vi "Set Control Appearance.vi"(4 "DigNum Refnum 2":refnum<vi>, 5 "DigNum Refnum":refnum<vi>, 6 "Bool Refnum":refnum<vi>, 7 "Arr Refnum":refnum<vi>, 8 "error in (no error)":errorcluster, 9 "Slide Refnum":refnum<vi>, 10 "Data In":T3, 11 "Display State In":T2 caption="State" {"# of Loops" min=1 step=1; "Index" min=0 step=1; "Program"."Step" min=0.001 max=80.0 step=0.001 format="%.2f"; "Program"."Target" format="%.2f"}) -> (0 "error out":errorcluster, 2 "Data Out":T3 caption="Data In", 3 "Display State Out":T2 caption="State" {"# of Loops" min=1 step=1; "Index" min=0 step=1; "Program"."Step" min=0.001 max=80.0 step=0.001 format="%.2f"; "Program"."Target" format="%.2f"})   [LabVIEW 2012, in "Multi Segment Waveform.xctl"]
doc: "Based on the current XControl state, set the appearance of the facade controls"
uses:
  Multi Segment Waveform.xctl
  State.ctl
  Data.ctl
  <vilib>/_xctls/Container State.ctl
  <vilib>/_xctls/XControlSupport.lvlib
panel:
  in  "Container State":T1
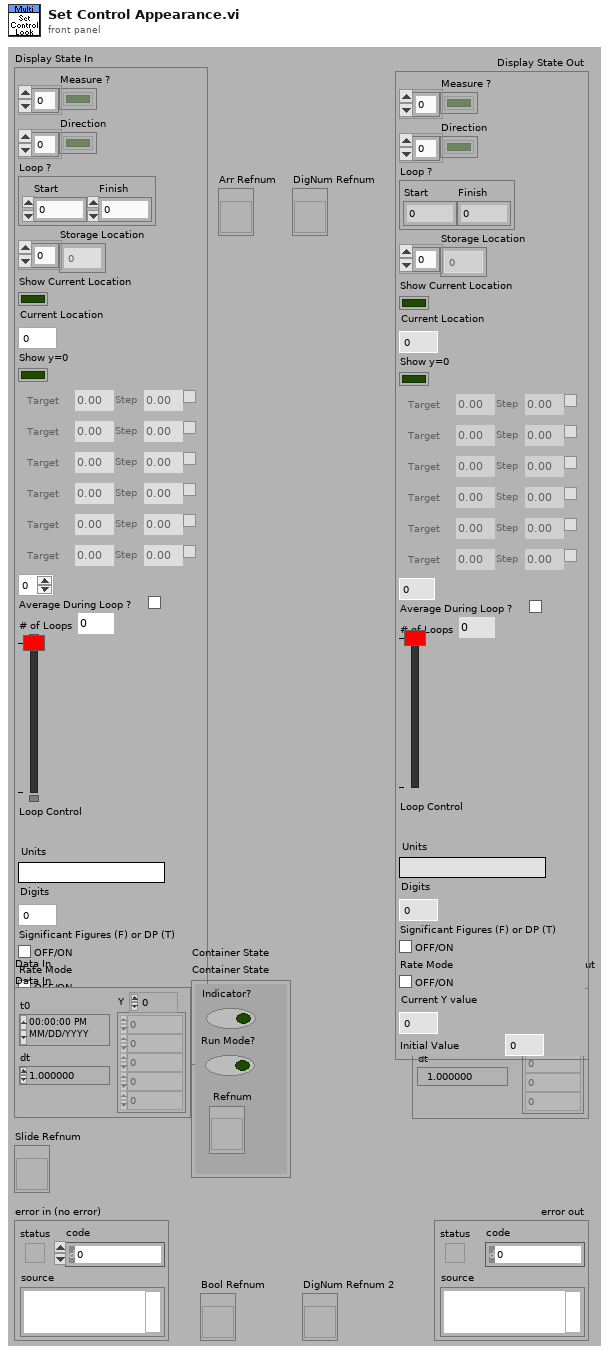
[diagram p1: front panel]
types:
  T1 = typedef "XControlSupport.lvlib/Container State.ctl" = cluster{"Indicator?":bool, "Run Mode?":bool, " Refnum":refnum<vi>}
  T2 = typedef "Multi Segment Waveform.xctl/State.ctl" = cluster{"Measure ?":bool[], "Direction":bool[], "Loop ?":cluster{"Start":i32, "Finish":i32}, "Storage Location":i32[], "Show Current Location":bool, "Current Location":i32, "Show y=0":bool, "Program":cluster{"Target":dbl, "Step":dbl, "Measure ?":bool}[], "Index":i32, "Average During Loop ?":bool, "# of Loops":u32, "Loop Control":cluster{i32, i32}, "Units":string, "Digits":i32, "Significant Figures (F) or DP (T)":bool, "Rate Mode":bool, "Current Y value":dbl, "Initial Value":dbl}
  T3 = typedef "Multi Segment Waveform.xctl/Data.ctl" = waveform(dbl)
  T4 = cluster{"Target":dbl, "Step":dbl, "Measure ?":bool}[]
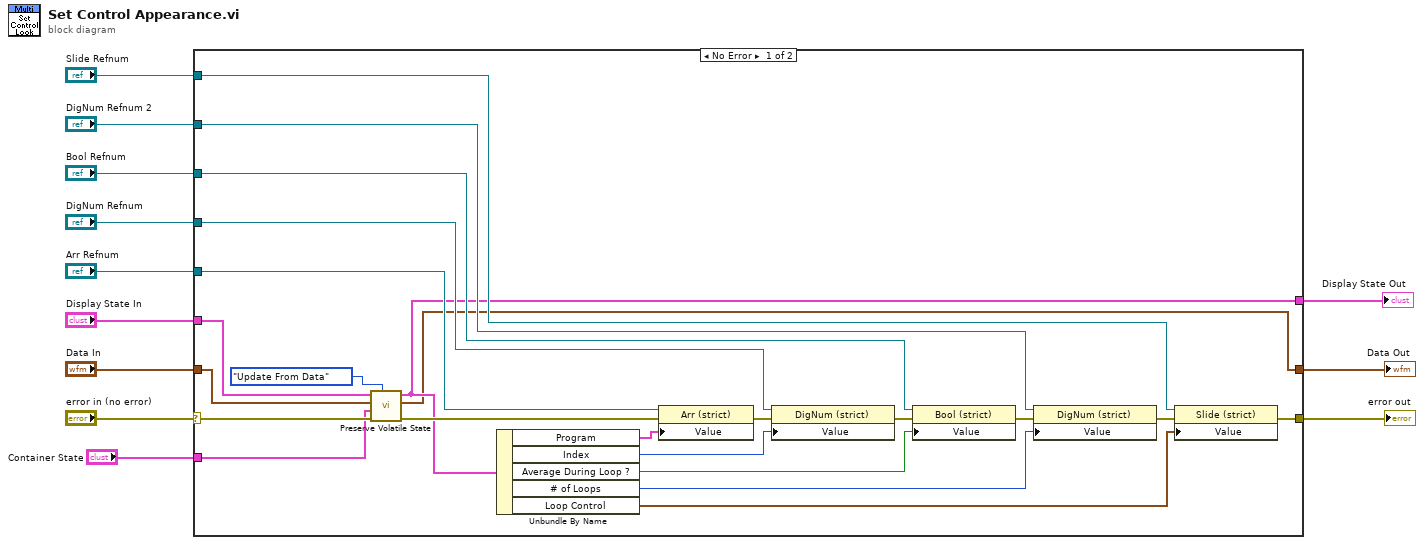
[diagram p0: block diagram]
diagram:
  n1 = case shown="No Error" "error in (no error)" {
    selector: "error in (no error)" -> [w18 w37]
    tunnel: [w35 w37] -> w11
    tunnel: "Display State In" -> [w19 _]
    tunnel: [w15 w36] -> w9
    tunnel: "Data In" -> [w20 w36]
    tunnel: "Arr Refnum" -> [w25 _]
    tunnel: "DigNum Refnum" -> [w24 _]
    tunnel: "Bool Refnum" -> [w23 _]
    tunnel: "DigNum Refnum 2" -> [w22 _]
    tunnel: "Slide Refnum" -> [w21 _]
    tunnel: [w16 _] -> w2
    tunnel: "Container State" -> [w13 _]
    frame No Error {
      n2 = call "Preserve Volatile State.vi"("Operation"=enum16{"Read", "Write", "Update From Data"}."Update From Data", "error in (no error)"=w18, "Container State"=w13, "Waveform"=w20, "Waveform State In"=w19) -> ("error out"=w17:errorcluster, "Waveform Out"=w15:T3, "Waveform State Out"=w16:T2)  [unwired: 4 out]
      n3 = Unbundle By Name(w16) -> ("Program"=w26:T4, "Index"=w28:i32, "Average During Loop ?"=w30:bool, "# of Loops"=w32:u32, "Loop Control"=w34:cluster{i32, i32})
      n4 = property on="Property Node" class="Arr (strict)"(reference=w25, error in=w17, "Value"=w26) -> (error out=w27:errorcluster)  [unwired: 1 out]
      n5 = property on="Property Node" class="DigNum (strict)"(reference=w24, error in=w27, "Value"=w28) -> (error out=w29:errorcluster)  [unwired: 1 out]
      n6 = property on="Property Node" class="Bool (strict)"(reference=w23, error in=w29, "Value"=w30) -> (error out=w31:errorcluster)  [unwired: 1 out]
      n7 = property on="Property Node" class="DigNum (strict)"(reference=w22, error in=w31, "Value"=w32) -> (error out=w33:errorcluster)  [unwired: 1 out]
      n8 = property on="Property Node" class="Slide (strict)"(reference=w21, error in=w33, "Value"=w34) -> (error out=w35:errorcluster)  [unwired: 1 out]
    }
    frame Error {
    }
  }
  "error out" <- w11
  "Data Out" <- w9
  "Display State Out" <- w2
